vi "1_Home_u_1.vi"() -> ()   [LabVIEW 2011]
uses:
  Globals/Global Recipe.vi
  Globals/Global VI.vi
panel:
  in  "Bank C Select All":bool caption="Bank"
  in  "Bank B Select All":bool caption="Bank"
  in  "Bank A Select All":bool caption="Bank A"
  in  "Bank B":bool[][](array[boolean])
  in  "Bank C":bool[][](array[boolean])
  in  "Bank A":bool[][](array[boolean])
  out "Run Status":bool
  in  "Stop Button":bool
  in  "Pause Button":bool
  in  "Play Button":bool
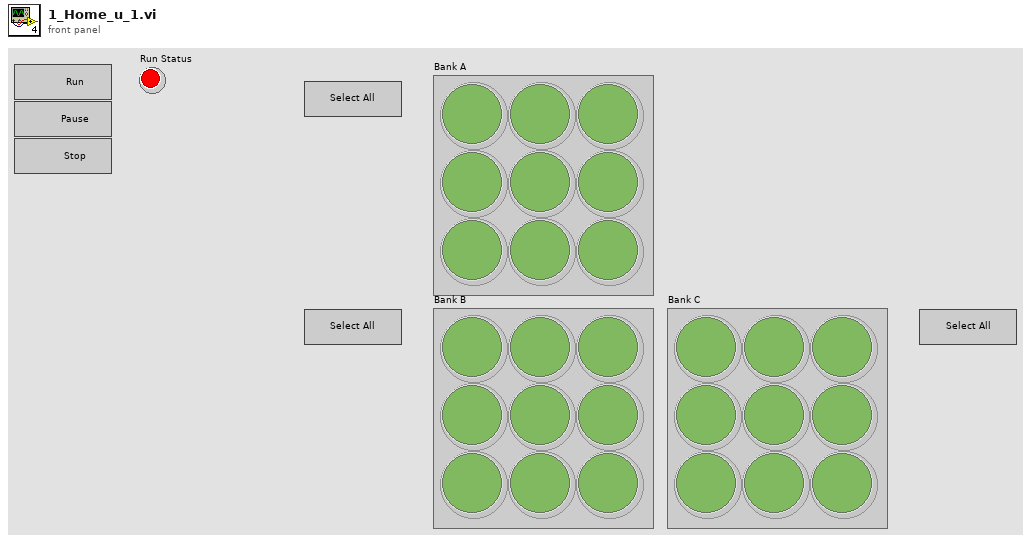
[diagram p1: front panel]
types:
  T1 = enum8{"Enabled", "Disabled", "Disabled and Grayed Out"}
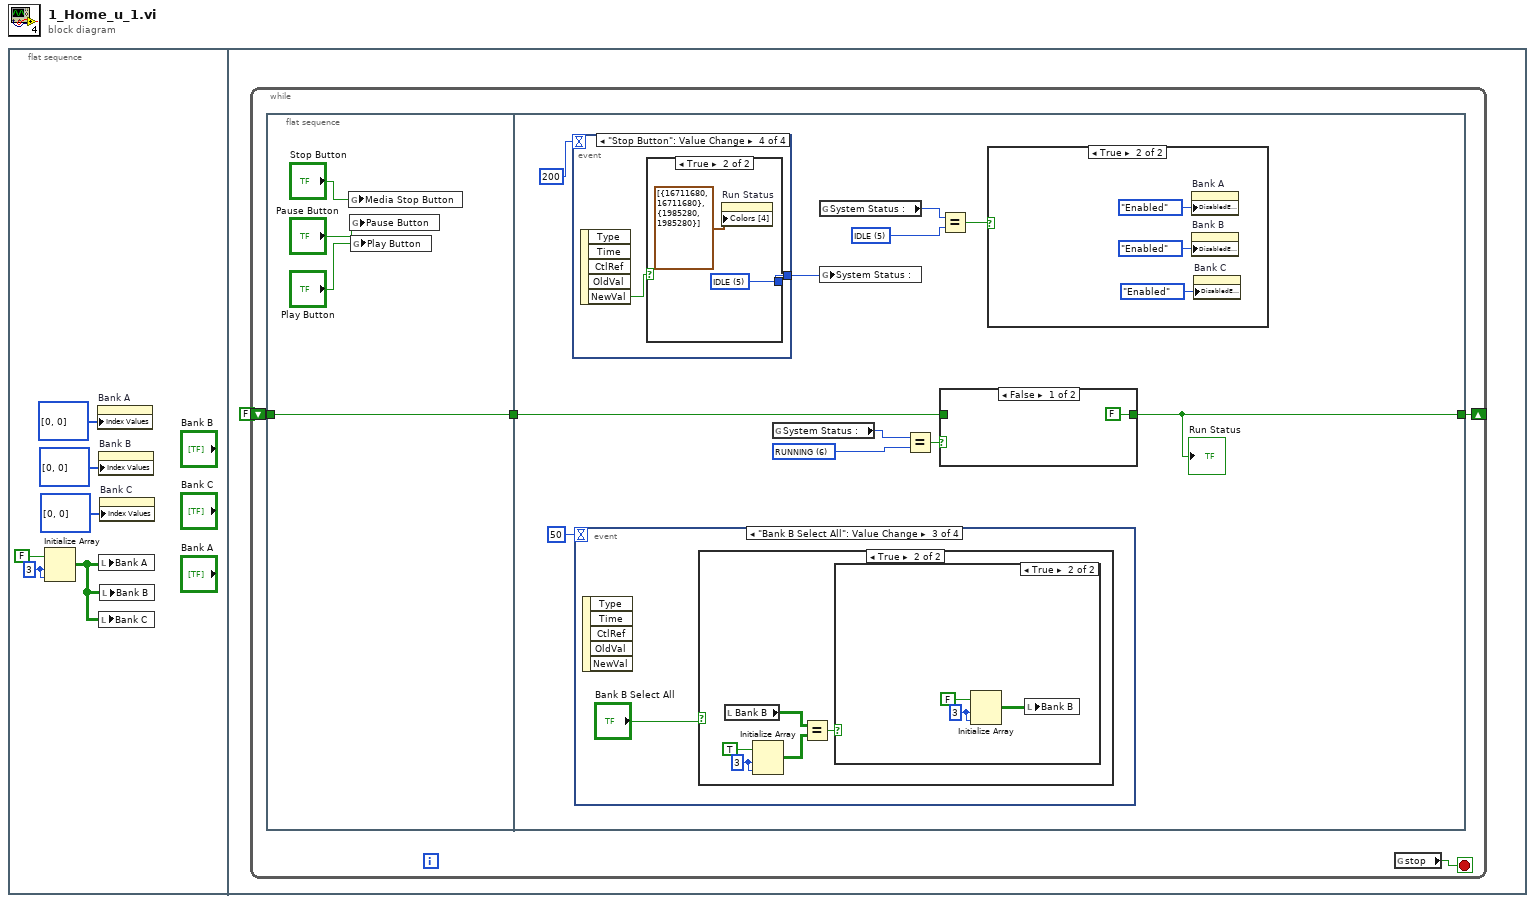
[diagram p0: block diagram]
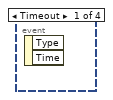
[diagram p2: hidden frame]
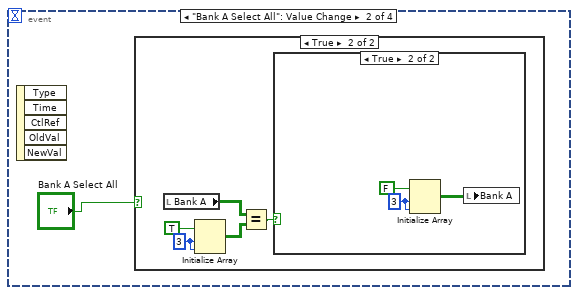
[diagram p3: hidden frame]
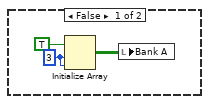
[diagram p5: hidden frame]
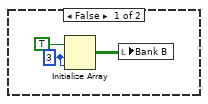
[diagram p7: hidden frame]
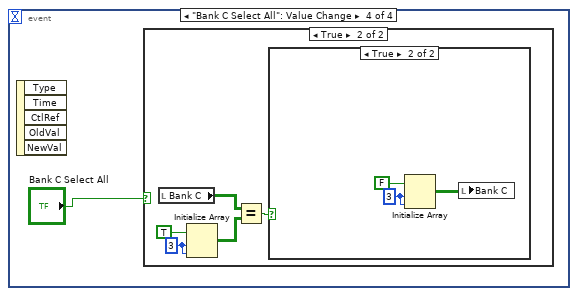
[diagram p8: hidden frame]
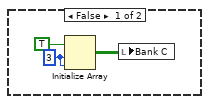
[diagram p10: hidden frame]
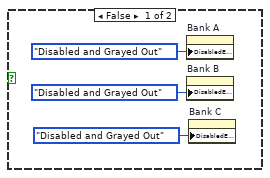
[diagram p11: hidden frame]
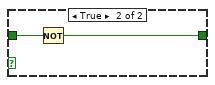
[diagram p12: hidden frame]
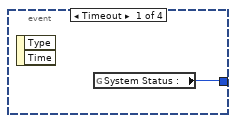
[diagram p13: hidden frame]
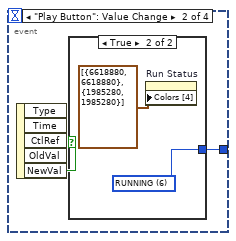
[diagram p14: hidden frame]
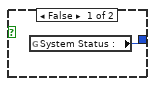
[diagram p15: hidden frame]
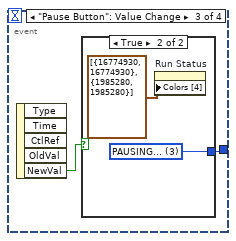
[diagram p16: hidden frame]
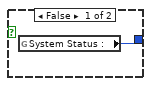
[diagram p17: hidden frame]
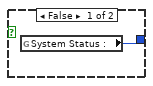
[diagram p18: hidden frame]
diagram:
  n1 = flat-sequence {
    frame #0 {
      w2 = 3 ("dimension size")
      n2 = Initialize Array(FALSE, w2, w2) -> (w1:bool[][])
      n3 = property on="Bank A" class="Arr (strict)"("Index Values"=u32[] [0, 0]) -> ()  [unwired: 2 in, 2 out]
      n4 = property on="Bank B" class="Arr (strict)"("Index Values"=u32[] [0, 0]) -> ()  [unwired: 2 in, 2 out]
      n5 = local write "Bank A"(w1) -> ()
      n6 = local write "Bank C"(w1) -> ()
      n7 = property on="Bank C" class="Arr (strict)"("Index Values"=u32[] [0, 0]) -> ()  [unwired: 2 in, 2 out]
      n8 = local write "Bank B"(w1) -> ()
    }
    frame #1 {
      n9 = while {
        shift-right: [w10] -> _
        shift-left: FALSE -> [w9]
        stop <- w11 stop-if-true
        n10 = flat-sequence {
          tunnel: w9 -> [w12]
          tunnel: [w12] -> w8
          tunnel: [w21] -> w10
          tunnel: w8 -> [w23]
          frame #0 {
            n11 = global write "Global Recipe.vi" "Media Stop Button"("Stop Button") -> ()
            n12 = global write "Global Recipe.vi" "Pause Button"("Pause Button") -> ()
            n13 = global write "Global Recipe.vi" "Play Button"("Play Button") -> ()
          }
          frame #1 {
            w18 = u16 5 items=["NOT READY", "E-STOPPED", "FAULTED", "PAUSING...", "PAUSED", "IDLE", "RUNNING", "UNCALIBRATED", "CALIBRATING...", "POWER OFF", "POWERING ON...", "MANUAL MODE", "CONNECTING..."] ("System Status :")
            w24 = u16 6 items=["NOT READY", "E-STOPPED", "FAULTED", "PAUSING...", "PAUSED", "IDLE", "RUNNING", "UNCALIBRATED", "CALIBRATING...", "POWER OFF", "POWERING ON...", "MANUAL MODE", "CONNECTING..."] ("System Status :")
            n14 = event shown="[3] \"Stop Button\": Value Change" {
              selector: _ -> [_ _ _ _]
              dyn-events: _ -> [_ _ _ _]
              timeout: 200 -> [_ _ _ _]
              tunnel: [w72 w73 w78 w83] -> w26
              event Timeout {
                n15 = event-data() -> ()  [unwired: 1 in, 2 out]
                n16 = global read "Global Recipe.vi" "System Status :"() -> (w72:u16)
              }
              event "Play Button": Value Change {
                n17 = event-data() -> ("NewVal"=w74:bool)  [unwired: 1 in, 4 out]
                n18 = case shown="True" w74 {
                  tunnel: [w75 w77] -> w73
                  frame False {
                    n19 = global read "Global Recipe.vi" "System Status :"() -> (w75:u16)
                  }
                  frame True {
                    w77 = u16 6 items=["NOT READY", "E-STOPPED", "FAULTED", "PAUSING...", "PAUSED", "IDLE", "RUNNING", "UNCALIBRATED", "CALIBRATING...", "POWER OFF", "POWERING ON...", "MANUAL MODE", "CONNECTING..."] ("System Status :")
                    n20 = property on="Run Status" class="Bool (strict)"("Colors [4]"=cluster{u32, u32}[] [{6618880, 6618880}, {1985280, 1985280}]) -> ()  [unwired: 2 in, 2 out]
                  }
                }
              }
              event "Pause Button": Value Change {
                n21 = event-data() -> ("NewVal"=w79:bool)  [unwired: 1 in, 4 out]
                n22 = case shown="True" w79 {
                  tunnel: [w80 w82] -> w78
                  frame False {
                    n23 = global read "Global Recipe.vi" "System Status :"() -> (w80:u16)
                  }
                  frame True {
                    w82 = u16 3 items=["NOT READY", "E-STOPPED", "FAULTED", "PAUSING...", "PAUSED", "IDLE", "RUNNING", "UNCALIBRATED", "CALIBRATING...", "POWER OFF", "POWERING ON...", "MANUAL MODE", "CONNECTING..."] ("System Status :")
                    n24 = property on="Run Status" class="Bool (strict)"("Colors [4]"=cluster{u32, u32}[] [{16774930, 16774930}, {1985280, 1985280}]) -> ()  [unwired: 2 in, 2 out]
                  }
                }
              }
              event "Stop Button": Value Change {
                n25 = event-data() -> ("NewVal"=w84:bool)  [unwired: 1 in, 4 out]
                n26 = case shown="True" w84 {
                  tunnel: [w85 w87] -> w83
                  frame False {
                    n27 = global read "Global Recipe.vi" "System Status :"() -> (w85:u16)
                  }
                  frame True {
                    w87 = u16 5 items=["NOT READY", "E-STOPPED", "FAULTED", "PAUSING...", "PAUSED", "IDLE", "RUNNING", "UNCALIBRATED", "CALIBRATING...", "POWER OFF", "POWERING ON...", "MANUAL MODE", "CONNECTING..."] ("System Status :")
                    n28 = property on="Run Status" class="Bool (strict)"("Colors [4]"=cluster{u32, u32}[] [{16711680, 16711680}, {1985280, 1985280}]) -> ()  [unwired: 2 in, 2 out]
                  }
                }
              }
            }
            n29 = event shown="[2] \"Bank B Select All\": Value Change" {
              selector: _ -> [_ _ _ _]
              dyn-events: _ -> [_ _ _ _]
              timeout: 50 -> [_ _ _ _]
              event Timeout {
                n30 = event-data() -> ()  [unwired: 1 in, 2 out]
              }
              event "Bank A Select All": Value Change {
                n31 = event-data() -> ()  [unwired: 1 in, 5 out]
                n32 = case shown="True" "Bank A Select All" {
                  frame False {
                  }
                  frame True {
                    w29 = 3 ("dimension size")
                    n33 = local read "Bank A"() -> (w31:bool[][])
                    n34 = Initialize Array(TRUE, w29, w29) -> (w32:bool[][])
                    n35 = Equal?(x=w31, y=w32) -> (x = y?=w28:bool)
                    n36 = case shown="True" w28 {
                      frame False {
                        w34 = 3 ("dimension size")
                        n37 = Initialize Array(TRUE, w34, w34) -> (w33:bool[][])
                        n38 = local write "Bank A"(w33) -> ()
                      }
                      frame True {
                        w37 = 3 ("dimension size")
                        n39 = Initialize Array(FALSE, w37, w37) -> (w36:bool[][])
                        n40 = local write "Bank A"(w36) -> ()
                      }
                    }
                  }
                }
              }
              event "Bank B Select All": Value Change {
                n41 = event-data() -> ()  [unwired: 1 in, 5 out]
                n42 = case shown="True" "Bank B Select All" {
                  frame False {
                  }
                  frame True {
                    w41 = 3 ("dimension size")
                    n43 = local read "Bank B"() -> (w43:bool[][])
                    n44 = Initialize Array(TRUE, w41, w41) -> (w44:bool[][])
                    n45 = Equal?(x=w43, y=w44) -> (x = y?=w40:bool)
                    n46 = case shown="True" w40 {
                      frame False {
                        w46 = 3 ("dimension size")
                        n47 = Initialize Array(TRUE, w46, w46) -> (w45:bool[][])
                        n48 = local write "Bank B"(w45) -> ()
                      }
                      frame True {
                        w49 = 3 ("dimension size")
                        n49 = Initialize Array(FALSE, w49, w49) -> (w48:bool[][])
                        n50 = local write "Bank B"(w48) -> ()
                      }
                    }
                  }
                }
              }
              event "Bank C Select All": Value Change {
                n51 = event-data() -> ()  [unwired: 1 in, 5 out]
                n52 = case shown="True" "Bank C Select All" {
                  frame False {
                  }
                  frame True {
                    w53 = 3 ("dimension size")
                    n53 = local read "Bank C"() -> (w55:bool[][])
                    n54 = Initialize Array(TRUE, w53, w53) -> (w56:bool[][])
                    n55 = Equal?(x=w55, y=w56) -> (x = y?=w52:bool)
                    n56 = case shown="True" w52 {
                      frame False {
                        w58 = 3 ("dimension size")
                        n57 = Initialize Array(TRUE, w58, w58) -> (w57:bool[][])
                        n58 = local write "Bank C"(w57) -> ()
                      }
                      frame True {
                        w61 = 3 ("dimension size")
                        n59 = Initialize Array(FALSE, w61, w61) -> (w60:bool[][])
                        n60 = local write "Bank C"(w60) -> ()
                      }
                    }
                  }
                }
              }
            }
            n61 = global read "Global Recipe.vi" "System Status :"() -> (w25:u16)
            n62 = global read "Global Recipe.vi" "System Status :"() -> (w17:u16)
            n63 = global write "Global Recipe.vi" "System Status :"(w26) -> ()
            n64 = Equal?(x=w25, y=w24) -> (x = y?=w22:bool)
            n65 = Equal?(x=w17, y=w18) -> (x = y?=w16:bool)
            n66 = case shown="False" w22 {
              tunnel: [FALSE w71] -> w21
              tunnel: w23 -> [_ w70]
              frame False {
              }
              frame True {
                n67 = Not(x=w70) -> (.not. x?=w71:bool)
              }
            }
            "Run Status" <- w21
            n68 = case shown="True" w16 {
              frame False {
                n69 = property on="Bank A" class="Arr (strict)"("DisabledEnum"=T1."Disabled and Grayed Out" ("Disabled")) -> ()  [unwired: 2 in, 2 out]
                n70 = property on="Bank B" class="Arr (strict)"("DisabledEnum"=T1."Disabled and Grayed Out" ("Disabled")) -> ()  [unwired: 2 in, 2 out]
                n71 = property on="Bank C" class="Arr (strict)"("DisabledEnum"=T1."Disabled and Grayed Out" ("Disabled")) -> ()  [unwired: 2 in, 2 out]
              }
              frame True {
                n72 = property on="Bank A" class="Arr (strict)"("DisabledEnum"=T1."Enabled" ("Disabled")) -> ()  [unwired: 2 in, 2 out]
                n73 = property on="Bank B" class="Arr (strict)"("DisabledEnum"=T1."Enabled" ("Disabled")) -> ()  [unwired: 2 in, 2 out]
                n74 = property on="Bank C" class="Arr (strict)"("DisabledEnum"=T1."Enabled" ("Disabled")) -> ()  [unwired: 2 in, 2 out]
              }
            }
          }
        }
        n75 = global read "Global VI.vi" "stop"() -> (w11:bool)
      }
    }
  }
